vi "controlAmplitude.vi"(7 "Set":bool, 8 "error in":errorcluster, 9 "amplitude [V] in":dbl, 10 "axis in":u8, 11 "connection ID":refnum<k5>) -> (0 "error out":errorcluster, 1 "amplitude [V] out":dbl, 2 "axis out":u8, 3 "connection ID":refnum<k5>)   [LabVIEW 2019]
panel:
  in  "Set Command":string="com.attocube.amc.control.setControlAmplitude"
  in  "Get Command":string="com.attocube.amc.control.getControlAmplitude"
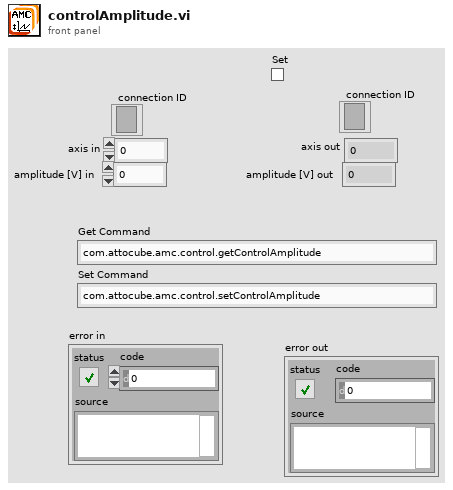
[diagram p1: front panel]
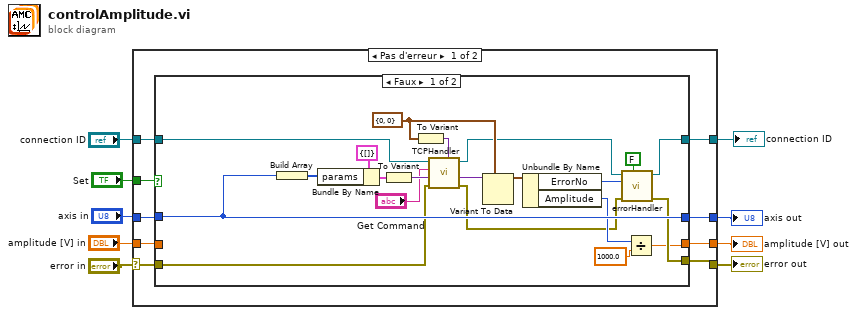
[diagram p0: block diagram]
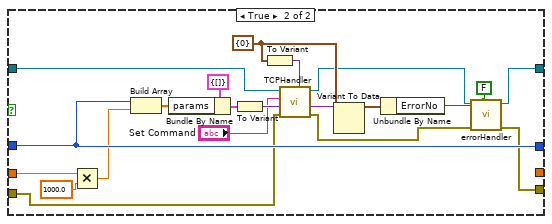
[diagram p2: hidden frame]
diagram:
  n1 = case shown="Pas d'erreur" "error in" {
    selector: "error in" -> [w10 w64]
    tunnel: "axis in" -> [w18 w63]
    tunnel: [w14 w64] -> w8
    tunnel: [w17 w63] -> w7
    tunnel: "amplitude [V] in" -> [w12 w61]
    tunnel: [w15 w61] -> w2
    tunnel: "Set" -> [w11 _]
    tunnel: [w13 w62] -> w5
    tunnel: "connection ID" -> [w16 w62]
    frame No Error {
      n2 = case shown="Faux" w11 {
        tunnel: [w22 w43] -> w13
        tunnel: w16 -> [w29 w55]
        tunnel: w18 -> [w31 w53]
        tunnel: [w31 w53] -> w17
        tunnel: [w24 _] -> w15
        tunnel: [w30 w50] -> w14
        tunnel: w12 -> [_ w45]
        tunnel: w10 -> [w19 w41]
        frame False {
          w27 = cluster{"ErrorNo":i16, "Amplitude":i64} {"ErrorNo"=0, "Amplitude"=0} ("input cluster")
          n3 = Build Array(w31) -> (w35:u8[])
          n4 = Bundle By Name(cluster=cluster{"params":i16[]} {"params"=[]} ("input cluster"), "params"=w35) -> (w36:cluster{"params":i16[]})
          n5 = To Variant(anything=w36) -> (Variant=w37:variant)
          n6 = To Variant(anything=w27) -> (Variant=w28:variant)
          n7 = call <userlib>:"TCPHandler.vi"("result Types"=w28, "error in (no error)"=w19, "params"=w37, "method"="Get Command", "connection ID"=w29) -> ("error out"=w20:errorcluster, "result"=w33:variant, "connection ID"=w23:refnum<k5>)  [unwired: 3 in, 1 out]
          n8 = Variant To Data(type=w27, Variant=w33) -> (data=w38:cluster{"ErrorNo":i16, "Amplitude":i64})  [unwired: 1 in, 1 out]
          n9 = Unbundle By Name(w38) -> ("ErrorNo"=w39:i16, "Amplitude"=w25:i64)
          n10 = call <userlib>:"errorHandler.vi"("show popup"=FALSE, "error in"=w20, "error number"=w39, "connection ID"=w23) -> ("error out"=w30:errorcluster, "connection ID"=w22:refnum<k5>)  [unwired: 6 in]
          n11 = Divide(x=w25, y=1000.0) -> (x/y=w24:dbl)
        }
        frame True {
          w48 = cluster{"ErrorNo":i16} {"ErrorNo"=0} ("input cluster")
          n12 = Multiply(x=w45, y=1000.0) -> (x*y=w46:dbl)
          n13 = Build Array(w53, w46) -> (w57:dbl[])
          n14 = Bundle By Name(cluster=cluster{"params":dbl[]} {"params"=[]} ("input cluster"), "params"=w57) -> (w56:cluster{"params":dbl[]})
          n15 = To Variant(anything=w56) -> (Variant=w54:variant)
          n16 = To Variant(anything=w48) -> (Variant=w49:variant)
          n17 = call <userlib>:"TCPHandler.vi"("result Types"=w49, "error in (no error)"=w41, "params"=w54, "method"="Set Command", "connection ID"=w55) -> ("error out"=w40:errorcluster, "result"=w59:variant, "connection ID"=w44:refnum<k5>)  [unwired: 3 in, 1 out]
          n18 = Variant To Data(type=w48, Variant=w59) -> (data=w52:cluster{"ErrorNo":i16})  [unwired: 1 in, 1 out]
          n19 = Unbundle By Name(w52) -> ("ErrorNo"=w51:i16)
          n20 = call <userlib>:"errorHandler.vi"("show popup"=FALSE, "error in"=w40, "error number"=w51, "connection ID"=w44) -> ("error out"=w50:errorcluster, "connection ID"=w43:refnum<k5>)  [unwired: 6 in]
        }
      }
    }
    frame Error {
    }
  }
  "error out" <- w8
  "axis out" <- w7
  "amplitude [V] out" <- w2
  "connection ID" <- w5
